vi "Read Parameters to process.vi"(8 "error in":errorcluster, 11 "Watchdog runtime in":refnum<class "Watchdog runtime.lvclass">) -> (0 "error out":errorcluster, 2 "Parameters to process":T1, 3 "Watchdog runtime out":refnum<class "Watchdog runtime.lvclass">)   [LabVIEW 2013, in "Watchdog runtime.lvclass"]
uses:
  Watchdog runtime.lvclass
  configuration/parameter data indices.ctl
  Watchdog runtime.lvclass/Watchdog runtime.ctl
  configuration/Watchdog configuration.lvclass
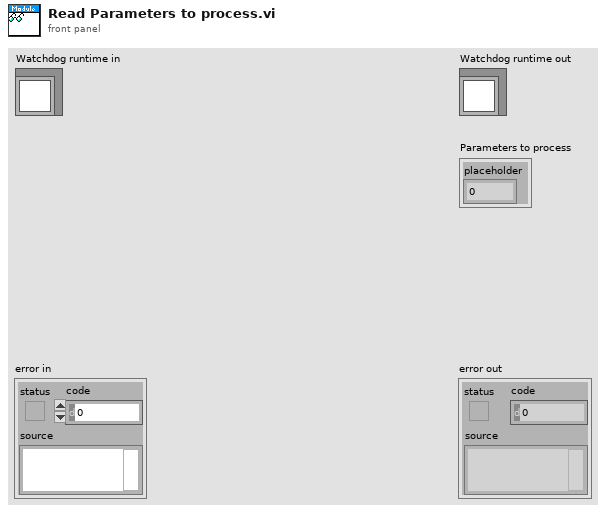
[diagram p1: front panel]
types:
  T1 = typedef "Watchdog configuration.lvclass/parameter data indices.ctl" = cluster{"placeholder":i32}
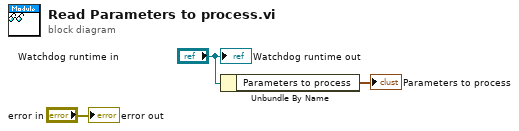
[diagram p0: block diagram]
diagram:
  n1 = Unbundle By Name("Watchdog runtime in") -> ("Parameters to process"=→"Parameters to process":T1)
  "error out" <- "error in"
  "Watchdog runtime out" <- "Watchdog runtime in"
